vi "export_DFX.vi"(0 "vacuum":sgl, 1 "Q1":sgl, 2 "P@Q1":sgl, 3 "Q2":sgl, 4 "P@Q2":sgl, 5 "Pmxax":sgl) -> ()   [LabVIEW 2012]
uses:
  FT_HMI.llb/GLOBAL_GEN.vi
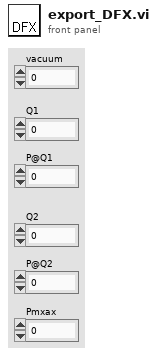
[diagram p1: front panel]
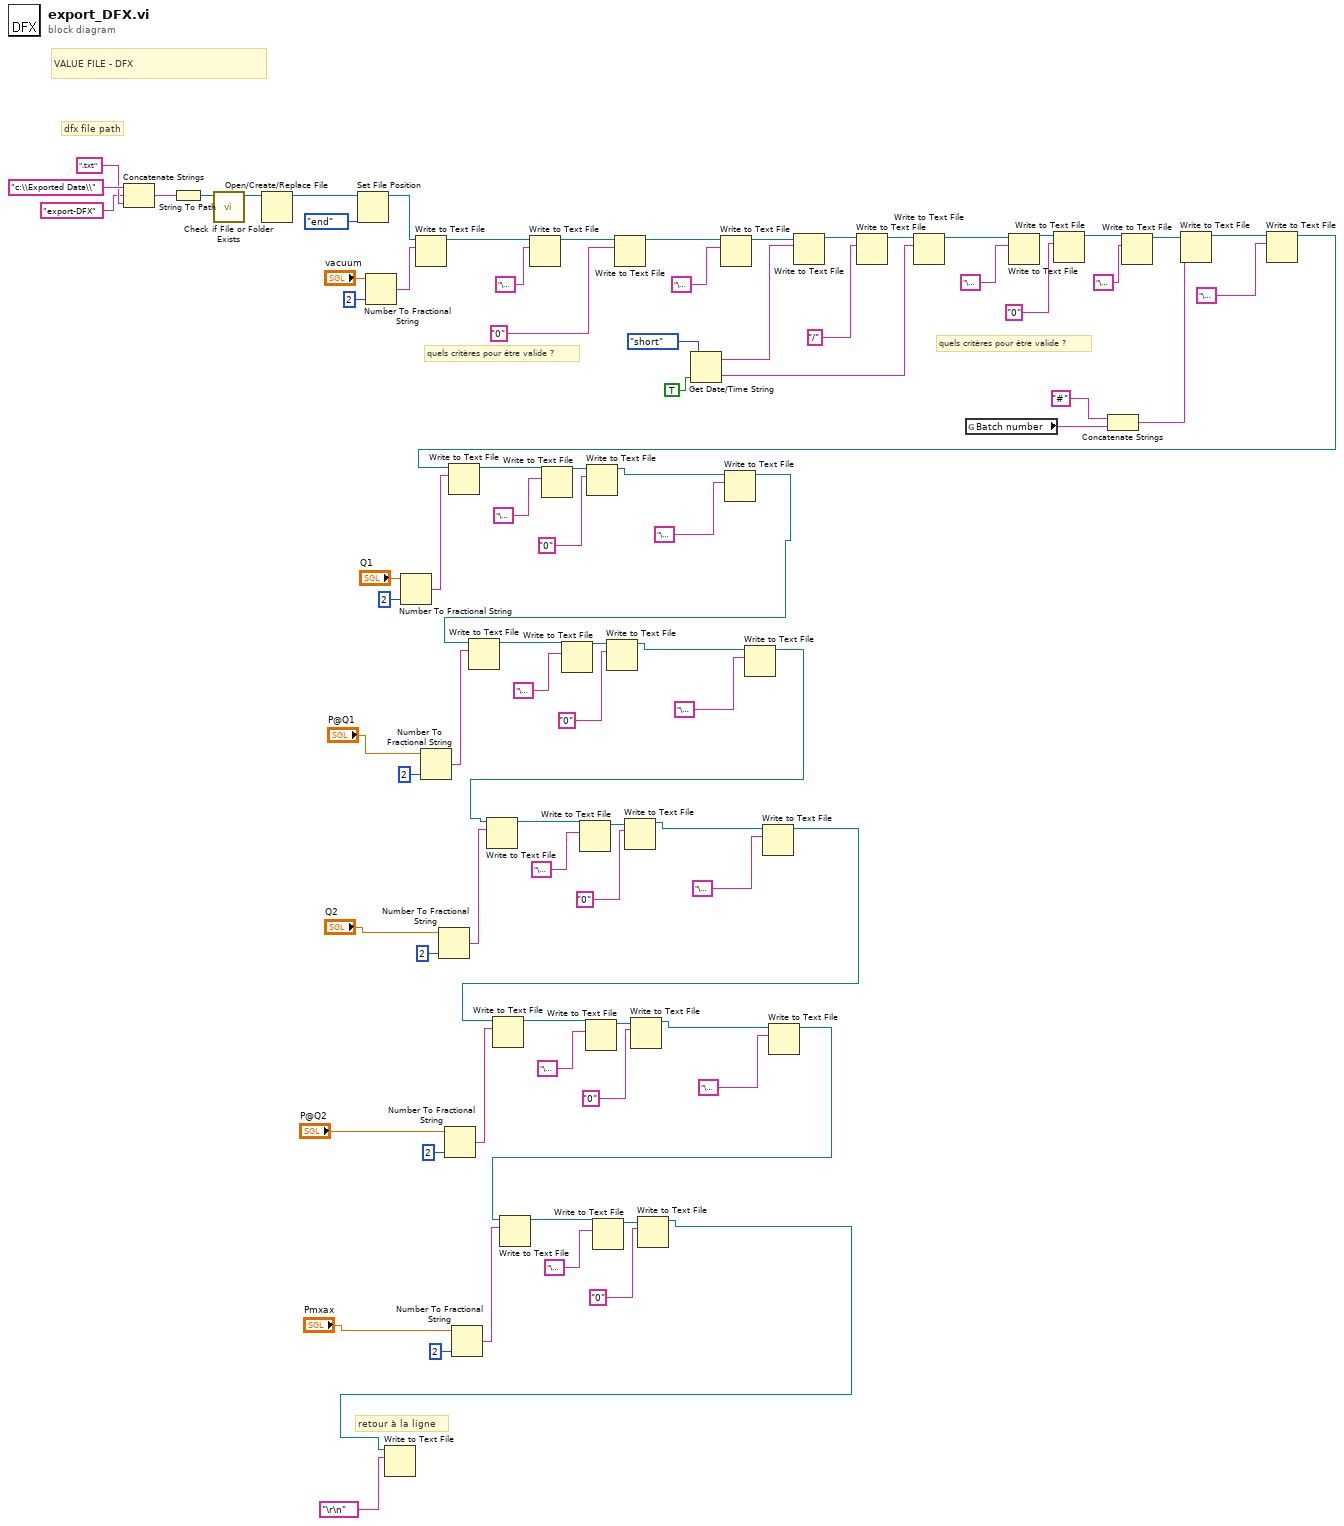
[diagram p0: block diagram]
diagram:
  # "quels critères pour être valide ?"
  # "dfx file path"
  # "VALUE FILE - DFX"
  # "quels critères pour être valide ?"
  # "retour à la ligne"
  n1 = Concatenate Strings("c:\\Exported Data\\", "export-DFX" ("string"), ".txt") -> (w85:string)
  n2 = String To Path(string=w85) -> (path=w87:path)
  n3 = call <vilib>:"Check if File or Folder Exists.vi"("path"=w87) -> ("dup path"=w59:path)  [unwired: 8 in, 2 out]
  n4 = Open/Create/Replace File(file path (use dialog)=w59) -> (refnum out=w57:refnum<file>)  [unwired: 5 in, 2 out]
  n5 = Set File Position(refnum=w57, from (0:start)=enum16{"start", "end", "current"}."end") -> (refnum out=w56:refnum<file>)  [unwired: 2 in, 1 out]
  n6 = Number To Fractional String(number="vacuum", precision (6)=i16 2 ("width (-)")) -> (F-format string=w60:string)  [unwired: 2 in]
  n7 = Number To Fractional String(number="Q1", precision (6)=i16 2 ("width (-)")) -> (F-format string=w49:string)  [unwired: 2 in]
  n8 = Write to Text File(file (use dialog)=w56, text=w60) -> (refnum out=w83:refnum<file>)  [unwired: 2 in, 2 out]
  n9 = Number To Fractional String(number="P@Q1", precision (6)=i16 2 ("width (-)")) -> (F-format string=w40:string)  [unwired: 2 in]
  n10 = Number To Fractional String(number="Q2", precision (6)=i16 2 ("width (-)")) -> (F-format string=w29:string)  [unwired: 2 in]
  n11 = Number To Fractional String(number="P@Q2", precision (6)=i16 2 ("width (-)")) -> (F-format string=w19:string)  [unwired: 2 in]
  n12 = Number To Fractional String(number="Pmxax", precision (6)=i16 2 ("width (-)")) -> (F-format string=w10:string)  [unwired: 2 in]
  n13 = Write to Text File(file (use dialog)=w83, text="\u0014") -> (refnum out=w80:refnum<file>)  [unwired: 2 in, 2 out]
  n14 = Write to Text File(file (use dialog)=w80, text="0") -> (refnum out=w79:refnum<file>)  [unwired: 2 in, 2 out]
  n15 = Get Date/Time String(date format (0)=enum16{"short", "long", "abbreviated"}."short", want seconds? (F)=TRUE) -> (date string=w75:string, time string=w74:string)  [unwired: 1 in]
  n16 = Write to Text File(file (use dialog)=w79, text="\u0014") -> (refnum out=w76:refnum<file>)  [unwired: 2 in, 2 out]
  n17 = Write to Text File(file (use dialog)=w76, text=w75) -> (refnum out=w71:refnum<file>)  [unwired: 2 in, 2 out]
  n18 = Write to Text File(file (use dialog)=w71, text="/") -> (refnum out=w70:refnum<file>)  [unwired: 2 in, 2 out]
  n19 = Write to Text File(file (use dialog)=w70, text=w74) -> (refnum out=w73:refnum<file>)  [unwired: 2 in, 2 out]
  n20 = global read "GLOBAL_GEN.vi" "Batch number"() -> (w66:string)
  n21 = Write to Text File(file (use dialog)=w73, text="\u0014") -> (refnum out=w67:refnum<file>)  [unwired: 2 in, 2 out]
  n22 = Write to Text File(file (use dialog)=w67, text="0") -> (refnum out=w51:refnum<file>)  [unwired: 2 in, 2 out]
  n23 = Concatenate Strings("#" ("string"), w66) -> (w64:string)
  n24 = Write to Text File(file (use dialog)=w51, text="\u0014") -> (refnum out=w50:refnum<file>)  [unwired: 2 in, 2 out]
  n25 = Write to Text File(file (use dialog)=w50, text=w64) -> (refnum out=w63:refnum<file>)  [unwired: 2 in, 2 out]
  n26 = Write to Text File(file (use dialog)=w63, text="\u000f") -> (refnum out=w30:refnum<file>)  [unwired: 2 in, 2 out]
  n27 = Write to Text File(file (use dialog)=w30, text=w49) -> (refnum out=w43:refnum<file>)  [unwired: 2 in, 2 out]
  n28 = Write to Text File(file (use dialog)=w43, text="\u0014") -> (refnum out=w44:refnum<file>)  [unwired: 2 in, 2 out]
  n29 = Write to Text File(file (use dialog)=w44, text="0") -> (refnum out=w41:refnum<file>)  [unwired: 2 in, 2 out]
  n30 = Write to Text File(file (use dialog)=w41, text="\u000f") -> (refnum out=w32:refnum<file>)  [unwired: 2 in, 2 out]
  n31 = Write to Text File(file (use dialog)=w32, text=w40) -> (refnum out=w35:refnum<file>)  [unwired: 2 in, 2 out]
  n32 = Write to Text File(file (use dialog)=w35, text="\u0014") -> (refnum out=w36:refnum<file>)  [unwired: 2 in, 2 out]
  n33 = Write to Text File(file (use dialog)=w36, text="0") -> (refnum out=w33:refnum<file>)  [unwired: 2 in, 2 out]
  n34 = Write to Text File(file (use dialog)=w33, text="\u000f") -> (refnum out=w23:refnum<file>)  [unwired: 2 in, 2 out]
  n35 = Write to Text File(file (use dialog)=w23, text=w29) -> (refnum out=w22:refnum<file>)  [unwired: 2 in, 2 out]
  n36 = Write to Text File(file (use dialog)=w22, text="\u0014") -> (refnum out=w21:refnum<file>)  [unwired: 2 in, 2 out]
  n37 = Write to Text File(file (use dialog)=w21, text="0") -> (refnum out=w20:refnum<file>)  [unwired: 2 in, 2 out]
  n38 = Write to Text File(file (use dialog)=w20, text="\u000f") -> (refnum out=w3:refnum<file>)  [unwired: 2 in, 2 out]
  n39 = Write to Text File(file (use dialog)=w3, text=w19) -> (refnum out=w14:refnum<file>)  [unwired: 2 in, 2 out]
  n40 = Write to Text File(file (use dialog)=w14, text="\u0014") -> (refnum out=w13:refnum<file>)  [unwired: 2 in, 2 out]
  n41 = Write to Text File(file (use dialog)=w13, text="0") -> (refnum out=w12:refnum<file>)  [unwired: 2 in, 2 out]
  n42 = Write to Text File(file (use dialog)=w12, text="\u000f") -> (refnum out=w2:refnum<file>)  [unwired: 2 in, 2 out]
  n43 = Write to Text File(file (use dialog)=w2, text=w10) -> (refnum out=w6:refnum<file>)  [unwired: 2 in, 2 out]
  n44 = Write to Text File(file (use dialog)=w6, text="\u0014") -> (refnum out=w5:refnum<file>)  [unwired: 2 in, 2 out]
  n45 = Write to Text File(file (use dialog)=w5, text="0") -> (refnum out=w1:refnum<file>)  [unwired: 2 in, 2 out]
  n46 = Write to Text File(file (use dialog)=w1, text="\r\n") -> ()  [unwired: 2 in, 3 out]
